vi "Build Draw Vectors.vi"(11 "Data Cluster":T1) -> (3 "Current CNV":dbl[](array[numeric]))   [LabVIEW 2019, in "CML UI.lvlib"]
uses:
  CML UI.lvlib
  Module Data--cluster.ctl
  Acquisition State.ctl
  Measurement UI Displays.ctl
  <vilib>/Analysis/3filter.llb/Filter Passband Type.ctl
  <vilib>/Analysis/baseanly.llb/Mean (DBL).vi
  <vilib>/Analysis/3filter.llb/Butterworth Filter (DBL).vi
  <vilib>/Analysis/NI_AALBase.lvlib
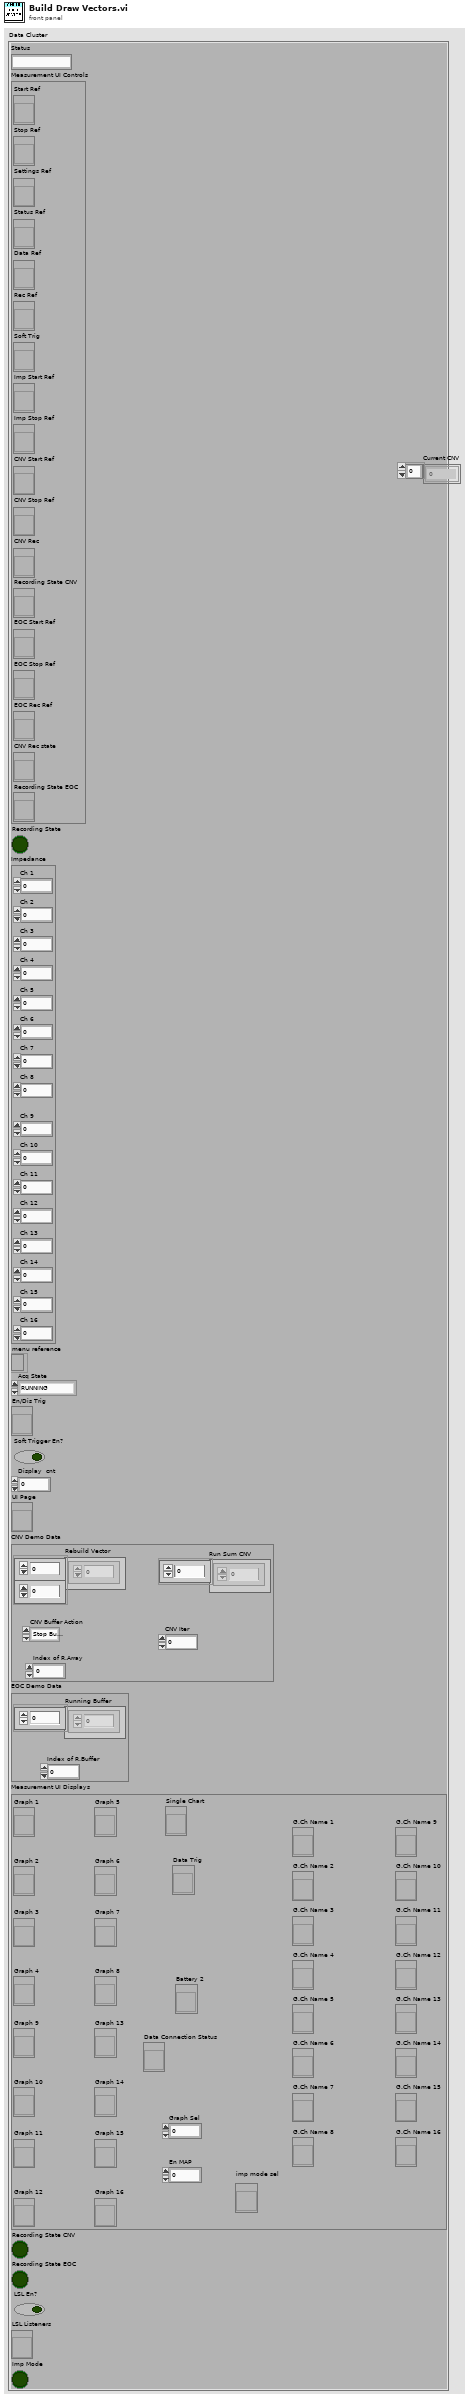
[diagram p1: front panel]
types:
  T1 = typedef "CML UI.lvlib/Module Data--cluster.ctl" = cluster{"Status":string, "Measurement UI Controls":cluster{"Start Ref":refnum<vi>, "Stop Ref":refnum<vi>, "Settings Ref":refnum<vi>, "Status Ref":refnum<vi>, "Data Ref":refnum<vi>, "Rec Ref":refnum<vi>, "Soft Trig":refnum<vi>, "Imp Start Ref":refnum<vi>, "Imp Stop Ref":refnum<vi>, "CNV Start Ref":refnum<vi>, "CNV Stop Ref":refnum<vi>, "CNV Rec":refnum<vi>, "Recording State CNV":refnum<vi>, "EOC Start Ref":refnum<vi>, "EOC Stop Ref":refnum<vi>, "EOC Rec Ref":refnum<vi>, "CNV Rec state":refnum<vi>, "Recording State EOC":refnum<vi>}, "Recording State":bool, "Impedance":cluster{"Ch 1":dbl, "Ch 2":dbl, "Ch 3":dbl, "Ch 4":dbl, "Ch 5":dbl, "Ch 6":dbl, "Ch 7":dbl, "Ch 8":dbl, "Ch 9":dbl, "Ch 10":dbl, "Ch 11":dbl, "Ch 12":dbl, "Ch 13":dbl, "Ch 14":dbl, "Ch 15":dbl, "Ch 16":dbl}, "menu reference ":refnum<k9>, "Acq State":T2, "En/Dis Trig":refnum<vi>, "Soft Trigger En?":bool, "Display  cnt":u8, "UI Page":refnum<vi>, "CNV Demo Data":cluster{"Rebuild Vector":dbl[][], "CNV Buffer Action":enum16{"Stop Buffer Fill", "Start Buffer Fill", "Analyze Buffer"}, "Index of R.Array":u16, "Run Sum CNV":dbl[], "CNV Iter":u16}, "EOC Demo Data":cluster{"Running Buffer":dbl[], "Index of R.Buffer":u8}, "Measurement UI Displays":T3, "Recording State CNV":bool, "Recording State EOC":bool, "LSL En?":bool, "LSL Listeners":refnum<vi>, "Imp Mode":bool}
  T2 = typedef "CML UI.lvlib/Acquisition State.ctl" = enum16{"RUNNING", "IDLE"}
  T3 = typedef "CML UI.lvlib/Measurement UI Displays.ctl" = cluster{"Graph 1":refnum<vi>, "Graph 2":refnum<vi>, "Graph 3":refnum<vi>, "Graph 4":refnum<vi>, "Graph 5":refnum<vi>, "Graph 6":refnum<vi>, "Graph 7":refnum<vi>, "Graph 8":refnum<vi>, "Graph 9":refnum<vi>, "Graph 10":refnum<vi>, "Graph 11":refnum<vi>, "Graph 12":refnum<vi>, "Graph 13":refnum<vi>, "Graph 14":refnum<vi>, "Graph 15":refnum<vi>, "Graph 16":refnum<vi>, "Battery 2":refnum<vi>, "Data Trig":refnum<vi>, "Data Connection Status":refnum<vi>, "Graph Sel":u8, "En MAP":u16, "Single Chart":refnum<vi>, "G.Ch Name 1":refnum<vi>, "G.Ch Name 2":refnum<vi>, "G.Ch Name 3":refnum<vi>, "G.Ch Name 4":refnum<vi>, "G.Ch Name 5":refnum<vi>, "G.Ch Name 6":refnum<vi>, "G.Ch Name 7":refnum<vi>, "G.Ch Name 8":refnum<vi>, "G.Ch Name 9":refnum<vi>, "G.Ch Name 10":refnum<vi>, "G.Ch Name 11":refnum<vi>, "G.Ch Name 12":refnum<vi>, "G.Ch Name 13":refnum<vi>, "G.Ch Name 14":refnum<vi>, "G.Ch Name 15":refnum<vi>, "G.Ch Name 16":refnum<vi>, "imp mode sel":refnum<vi>}
  T4 = typedef "NI_AALBase.lvlib/Filter Passband Type.ctl" = enum32{"Lowpass", "Highpass", "Bandpass", "Bandstop"}
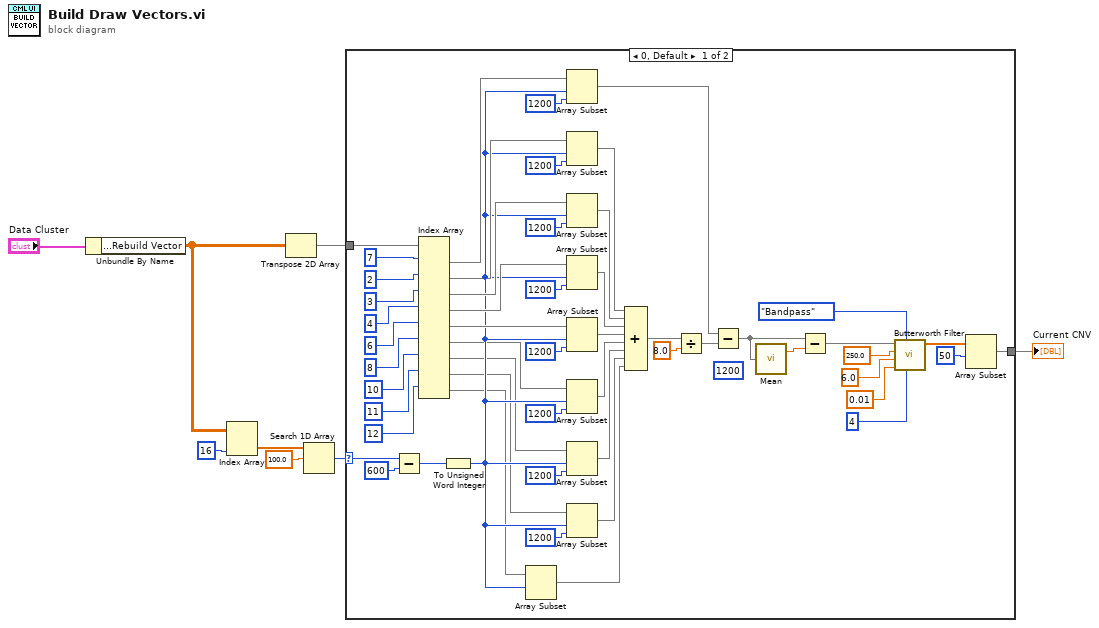
[diagram p0: block diagram]
diagram:
  n1 = Unbundle By Name("Data Cluster") -> ("CNV Demo Data.Rebuild Vector"=w2:dbl[][])
  n2 = Index Array(array=w2, index (col)=16 ("disabled index (col)")) -> (element=w8:dbl[])  [unwired: 1 in]
  n3 = Transpose 2D Array(2D array=w2) -> (transposed array=w1:dbl[][])
  n4 = Search 1D Array(1D array=w8, element=100.0) -> (index of element=w4:i32)  [unwired: 1 in]
  n5 = case shown="0, Default" w4 {
    selector: w4 -> [w61 _]
    tunnel: w1 -> [w62 _]
    tunnel: [w36 _] -> w3
    frame 0, Default {
      (unwired) 1200 ("length")
      n6 = Subtract(x=w61, y=600) -> (x-y=w59:i32)
      n7 = Index Array(array=w62, index (row) #1=7 ("disabled index (col)"), index (row) #2=2 ("index (row)"), index (row) #3=3 ("index (row)"), index (row) #4=4 ("index (row)"), index (row) #5=6 ("index (row)"), index (row) #6=8 ("index (row)"), index (row) #7=10 ("index (row)"), index (row) #8=11 ("index (row)"), index (row) #9=12 ("index (row)")) -> (element #1=w35:dbl[], element #2=w29:dbl[], element #3=w27:dbl[], element #4=w25:dbl[], element #5=w19:dbl[], element #6=w16:dbl[], element #7=w14:dbl[], element #8=w12:dbl[], element #9=w10:dbl[])  [unwired: 9 in]
      n8 = To Unsigned Word Integer(number=w59) -> (unsigned 16bit integer=w18:u16)
      n9 = Array Subset(array=w10, index=w18) -> (w9:dbl[])  [unwired: 1 in]
      n10 = Array Subset(array=w35, index=w18, length=1200) -> (w33:dbl[])
      n11 = Array Subset(array=w29, index=w18, length=1200) -> (w28:dbl[])
      n12 = Array Subset(array=w27, index=w18, length=1200) -> (w26:dbl[])
      n13 = Array Subset(array=w25, index=w18, length=1200) -> (w24:dbl[])
      n14 = Array Subset(array=w19, index=w18, length=1200) -> (w17:dbl[])
      n15 = Array Subset(array=w16, index=w18, length=1200) -> (w15:dbl[])
      n16 = Array Subset(array=w14, index=w18, length=1200) -> (w13:dbl[])
      n17 = Array Subset(array=w12, index=w18, length=1200) -> (w11:dbl[])
      n18 = Compound Arithmetic op=ADD(w28, w26, w24, w17, w15, w13, w11, w9) -> (w54:dbl[])
      n19 = Divide(x=w54, y=8.0) -> (x/y=w56:dbl[])
      n20 = Subtract(x=w33, y=w56) -> (x-y=w57:dbl[])
      n21 = call-poly <vilib>:"Mean.vi"("X"=w57) -> ("mean"=w58:dbl)  [unwired: 1 out]
      n22 = Subtract(x=w57, y=w58) -> (x-y=w37:dbl[])
      n23 = call-poly <vilib>:"Butterworth Filter.vi"("order"=4, "filter type"=Filter_Passband_Type."Bandpass", "low cutoff freq: fl"=0.01, "high cutoff freq: fh"=6.0, "sampling freq: fs"=250.0, "X"=w37) -> ("Filtered X"=w39:dbl[])  [unwired: 2 in, 1 out]
      n24 = Array Subset(array=w39, index=50) -> (w36:dbl[])  [unwired: 1 in]
    }
    frame -1 {
    }
  }
  "Current CNV" <- w3
